vi "WPILibNextRecord.vi"(8 "error in (no error)":errorcluster, 11 "Byte Stream File in":refnum<file>) -> (0 "error out":errorcluster, 2 "Record":T1, 3 "refnum out":refnum<file>)   [LabVIEW 2020]
uses:
  Typedef/Record.ctl
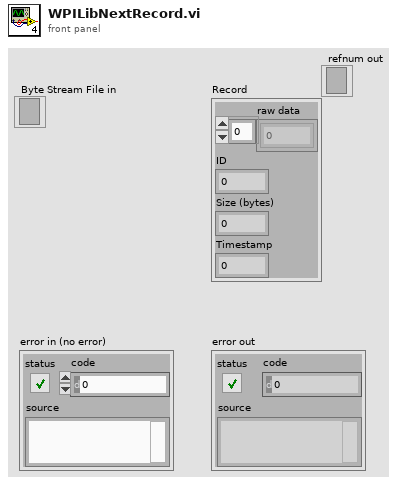
[diagram p1: front panel]
types:
  T1 = typedef "Record.ctl" = cluster{"raw data":u8[], "ID":u32, "Size (bytes)":u32, "Timestamp":u64}
  T2 = enum16{"big-endian, network order", "native, host order", "little-endian"}
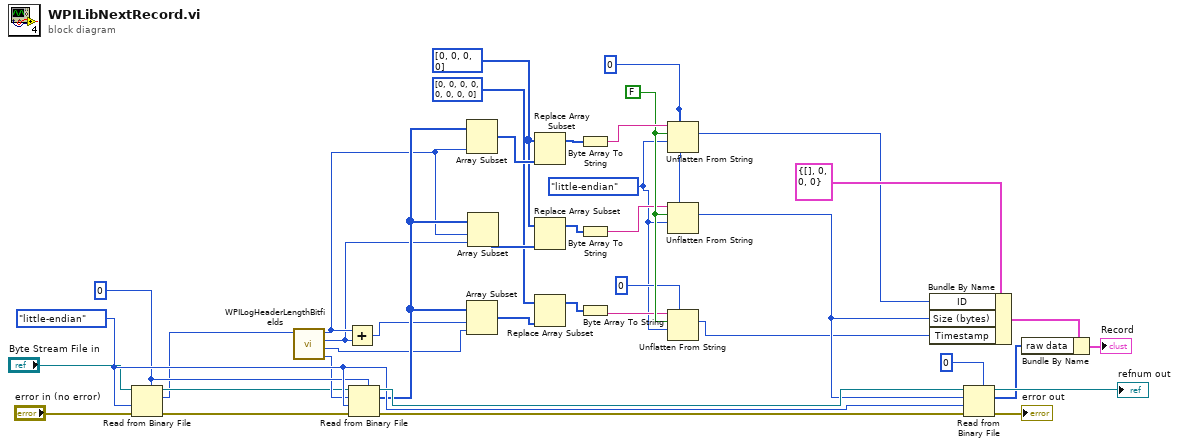
[diagram p0: block diagram]
diagram:
  w9 = T2."little-endian" ("byte order (0:big-endian, network order)")
  w11 = u32 0
  w14 = FALSE ("data includes array or string size? (T)")
  w21 = u8[] [0, 0, 0, 0]
  w31 = u8 0 ("Header Length Field")
  w36 = T2."little-endian" ("byte order (0:big-endian, network order)")
  n1 = Read from Binary File(5:w31, 8:"error in (no error)", 9:w36, 11:"Byte Stream File in") -> (0:w28:errorcluster, 2:w27:u8, 3:w29:refnum<file>)  [unwired: 2 in, 1 out]
  n2 = call "WPILogHeaderLengthBitfields.vi"("Header Length Field"=w27) -> ("Header Remainging Bytes"=w30:u8, "Timestamp Length"=w1:u8, "Payload Size Length"=w3:u8, "Entity ID Length"=w4:u8)  [unwired: 7 in]
  n3 = Add(x=w4, y=w3) -> (x+y=w2:u8)
  n4 = Read from Binary File(5:w31, 8:w28, 9:w36, 10:w30, 11:w29) -> (0:w35:errorcluster, 2:w32:u8[], 3:w37:refnum<file>)  [unwired: 1 in, 1 out]
  n5 = Array Subset(array=w32, length=w4) -> (w23:u8[])  [unwired: 1 in]
  n6 = Array Subset(array=w32, index=w2, length=w1) -> (w19:u8[])
  n7 = Array Subset(array=w32, index=w4, length=w3) -> (w22:u8[])
  n8 = Replace Array Subset(array=w21, new element=w23) -> (w18:u8[])  [unwired: 1 in]
  n9 = Replace Array Subset(array=w21, new element=w22) -> (w17:u8[])  [unwired: 1 in]
  n10 = Replace Array Subset(array=u8[] [0, 0, 0, 0, 0, 0, 0, 0], new element=w19) -> (w16:u8[])  [unwired: 1 in]
  n11 = Byte Array To String(unsigned byte array=w18) -> (string=w15:string)
  n12 = Byte Array To String(unsigned byte array=w17) -> (string=w13:string)
  n13 = Byte Array To String(unsigned byte array=w16) -> (string=w12:string)
  n14 = Unflatten From String(type=w11, binary string=w15, data includes array or string size? (T)=w14, byte order (0:big-endian, network order)=w9) -> (value=w8:u32)  [unwired: 1 in, 2 out]
  n15 = Unflatten From String(type=w11, binary string=w13, data includes array or string size? (T)=w14, byte order (0:big-endian, network order)=w9) -> (value=w7:u32)  [unwired: 1 in, 2 out]
  n16 = Unflatten From String(type=u64 0, binary string=w12, data includes array or string size? (T)=w14, byte order (0:big-endian, network order)=w9) -> (value=w6:u64)  [unwired: 1 in, 2 out]
  n17 = Bundle By Name(cluster=T1 {"raw data"=[], "ID"=0, "Size (bytes)"=0, "Timestamp"=0} ("Record"), "ID"=w8, "Size (bytes)"=w7, "Timestamp"=w6) -> (w34:T1)
  n18 = Read from Binary File(5:u8 0 ("Header Length Field"), 8:w35, 9:w36, 10:w7, 11:w37) -> (0:→"error out":errorcluster, 2:w5:u8[], 3:→"refnum out":refnum<file>)  [unwired: 1 in, 1 out]
  n19 = Bundle By Name(cluster=w34, "raw data"=w5) -> (→"Record":T1)
